vi "ParseArduinoHexPacket.vi"(11 "read buffer":string="01000000b88201005d603b4166f1b83f2a436d416f82b64159f3fa420000000000\n") -> (1 "Float Array":sgl[](array[numeric]), 2 "automatic":u8, 3 "start_of_packet":u8, 5 "Simulate Input":u8)   [LabVIEW 2014]
panel:
  out "substring 3":string
  out "substring 2":string
  out "substring":string
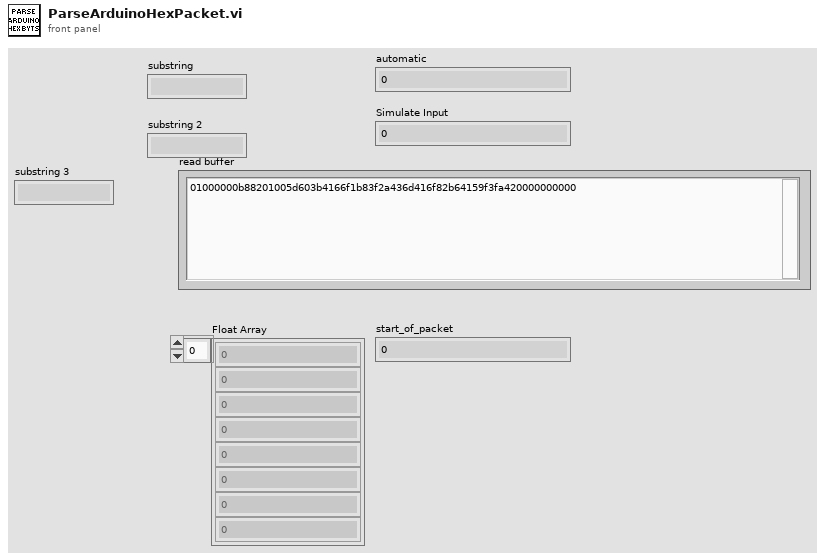
[diagram p1: front panel]
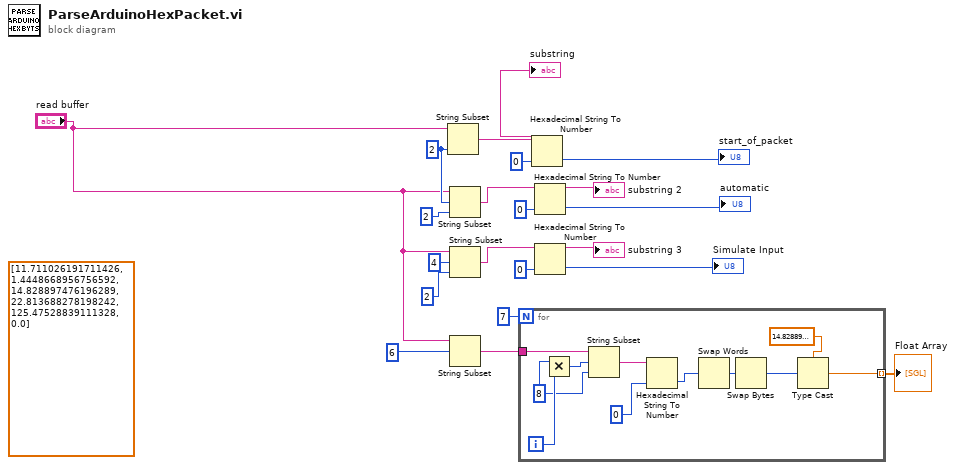
[diagram p0: block diagram]
diagram:
  (unwired) sgl[] [11.711026, 1.4448669, 14.828897, 22.813688, 125.47529, 0.0] ("Float Array")
  w16 = 2 ("length (rest)")
  n1 = String Subset(string="read buffer", length (rest)=w16) -> (substring=w18:string)  [unwired: 1 in]
  "substring" <- w18
  n2 = String Subset(string="read buffer", offset (0)=w16, length (rest)=2 ("length (rest)")) -> (substring=w14:string)
  "substring 2" <- w14
  n3 = String Subset(string="read buffer", offset (0)=4, length (rest)=2 ("length (rest)")) -> (substring=w5:string)
  "substring 3" <- w5
  n4 = String Subset(string="read buffer", offset (0)=6 ("length (rest)")) -> (substring=w11:string)  [unwired: 1 in]
  n5 = for {
    N: 7 -> [_]
    tunnel: w11 -> [w29]
    tunnel: [w19] -> w10 mode=indexing
    i -> [w27]
    w26 = 8 ("length (rest)")
    n6 = Multiply(x=w26, y=w27) -> (x*y=w28:i32)
    n7 = String Subset(string=w29, offset (0)=w28, length (rest)=w26) -> (substring=w25:string)
    n8 = Hexadecimal String To Number(string=w25, default (0uL)=0 ("default (0 U32)")) -> (number=w23:i32)  [unwired: 1 in, 1 out]
    n9 = Swap Words(1:w23) -> (0:w22:i32)
    n10 = Swap Bytes(anything=w22) -> (byte swapped=w21:i32)
    n11 = Type Cast(type=sgl 14.828897 ("Numeric"), x=w21) -> (*(type *) &x=w19:sgl)
  }
  "Float Array" <- w10
  n12 = Hexadecimal String To Number(string=w18, default (0uL)=u8 0 ("default (0 U32)")) -> (number=→"start_of_packet":u8)  [unwired: 1 in, 1 out]
  n13 = Hexadecimal String To Number(string=w14, default (0uL)=u8 0 ("default (0 U32)")) -> (number=→"automatic":u8)  [unwired: 1 in, 1 out]
  n14 = Hexadecimal String To Number(string=w5, default (0uL)=u8 0 ("default (0 U32)")) -> (number=→"Simulate Input":u8)  [unwired: 1 in, 1 out]
